vi "move.vi"(8 "error in (no error)":errorcluster, 11 "focus in":refnum<class "focus.lvclass">) -> (0 "error out":errorcluster, 3 "focus out":refnum<class "focus.lvclass">)   [LabVIEW 2012, in "focus.lvclass"]
uses:
  focus.lvclass
  focus.lvclass/focus.ctl
panel:
  out "Controller error":bool
  out "Target position":dbl[][](array[numeric])
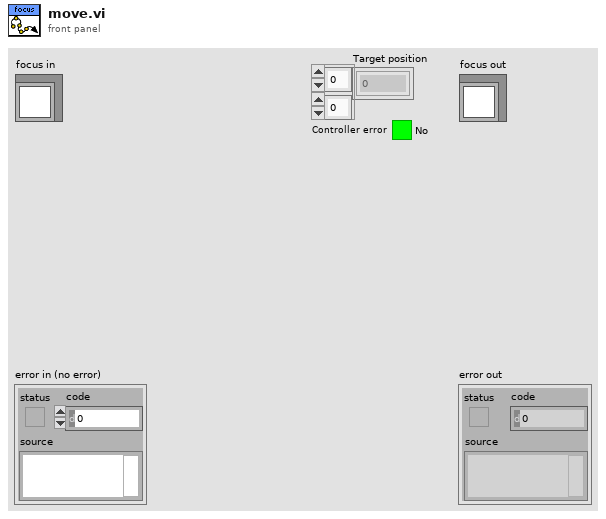
[diagram p1: front panel]
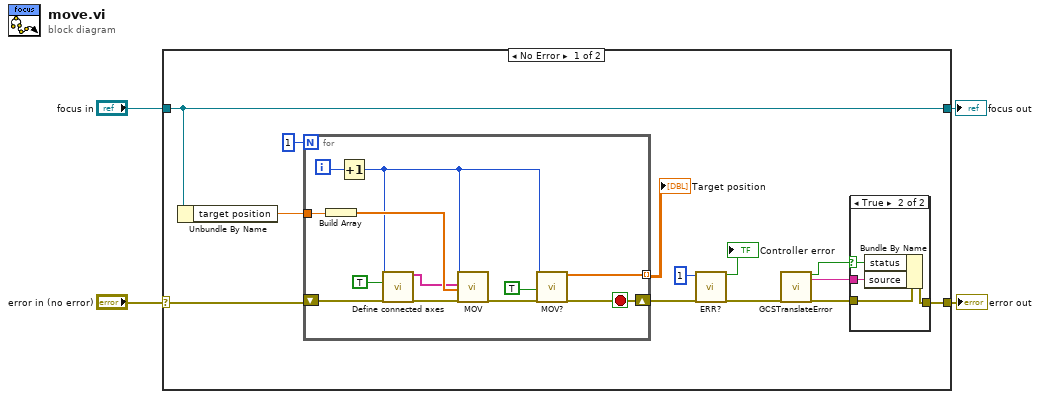
[diagram p0: block diagram]
diagram:
  n1 = case shown="No Error" "error in (no error)" {
    selector: "error in (no error)" -> [w14 w36]
    tunnel: [w7 w36] -> w3
    tunnel: [w17 w35] -> w1
    tunnel: "focus in" -> [w17 w35]
    frame No Error {
      n2 = Unbundle By Name(w17) -> ("target position"=w15:dbl)
      n3 = for {
        N: 1 -> [_]
        tunnel: w15 -> [w31]
        shift-right: [w24] -> w12
        shift-left: w14 -> [w33]
        tunnel: [w23] -> w13 mode=indexing
        i -> [w34]
        stop <- w24 stop-if-true
        n4 = Build Array(w31) -> (w30:dbl[])
        n5 = Increment(x=w34) -> (x+1=w25:i32)
        n6 = call "Define connected axes.vi"("System no."=w25, "Read from\ncontroller?"=TRUE ("Read from\ncontroller?"), "error in"=w33) -> ("Conn. Axes out"=w28:string[], "error out"=w29:errorcluster)  [unwired: 15 in]
        n7 = call "MOV.vi"("System no."=w25, "Axes to move"=w28, "Position values"=w30, "error in"=w29) -> ("error out"=w27:errorcluster)  [unwired: 15 in]
        n8 = call "MOV?.vi"("System no."=w25, "All axes?"=TRUE, "error in"=w27) -> ("Target position"=w23:dbl[], "error out"=w24:errorcluster)  [unwired: 15 in]
      }
      "Target position" <- w13
      n9 = call "ERR?.vi"("System no."=1, "error in"=w12) -> ("Controller error"=→"Controller error":bool, "error out"=w9:errorcluster)  [unwired: 16 in]
      n10 = call "GCSTranslateError.vi"("error in"=w9) -> ("GCS Error?"=w5:bool, "Error Description"=w6:string, "error out"=w8:errorcluster)  [unwired: 16 in]
      n11 = case shown="True" w5 {
        selector: w5 -> [_ w20]
        tunnel: w8 -> [w18 w22]
        tunnel: [w18 w21] -> w7
        tunnel: w6 -> [_ w19]
        frame False {
        }
        frame True {
          n12 = Bundle By Name(cluster=w22, "status"=w20, "source"=w19) -> (w21:errorcluster)
        }
      }
    }
    frame Error {
    }
  }
  "error out" <- w3
  "focus out" <- w1
